vi "Stop_acquisition.vi"(8 "error in (no error)":errorcluster, 11 ".NET Refnum in":refnum<k24>) -> (0 "error out":errorcluster, 3 ".NET Refnum out":refnum<k24>)   [LabVIEW 2021]
uses:
  C:/Program Files/Thorlabs/Scientific Imaging/ThorCam/uc480DotNet.dll
  Program Files/Thorlabs/Scientific Imaging/ThorCam/uc480DotNet.dll
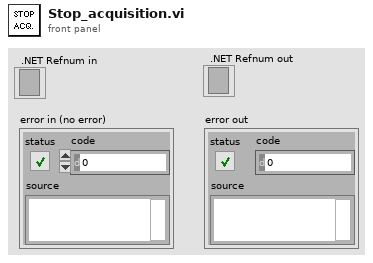
[diagram p1: front panel]
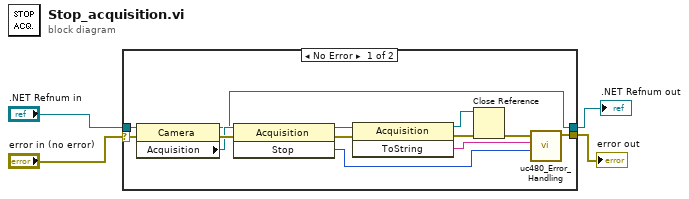
[diagram p0: block diagram]
diagram:
  n1 = case shown="No Error" "error in (no error)" {
    selector: "error in (no error)" -> [w6 w19]
    tunnel: ".NET Refnum in" -> [w14 w18]
    tunnel: [w7 w19] -> w3
    tunnel: [w5 w18] -> w1
    frame No Error {
      n2 = property class="Camera"(reference=w14, error in=w6) -> (reference out=w5:refnum<k24>, error out=w10:errorcluster, "Acquisition"=w9:refnum<k24>)
      n3 = invoke class="Acquisition" method="Stop"(reference=w9, error in=w10) -> (reference out=w12:refnum<k24>, error out=w11:errorcluster, "Stop"=w13:i32)  [unwired: 1 in]
      n4 = invoke class="Acquisition" method="ToString"(reference=w12, error in=w11) -> (reference out=w17:refnum<k24>, error out=w15:errorcluster, "ToString"=w8:string)  [unwired: 1 in]
      n5 = Close Reference(reference=w17, error in (no error)=w15) -> (error out=w16:errorcluster)
      n6 = call "uc480_Error_Handling.vi"("Error Code"=w13, "Error String"=w8, "Error In"=w16) -> ("Error Out"=w7:errorcluster)  [unwired: 8 in]
    }
    frame Error {
    }
  }
  "error out" <- w3
  ".NET Refnum out" <- w1
